vi "Computer_GUI_2.vi"(11 "GUI_cluster":T1={"Sub Panel"=refnum, "GUIdevice"="Bella_LP_Mode", "CtlRef"=refnum, "user event out"=refnum}) -> ()   [LabVIEW 2011]
uses:
  GUI_Template/GUI_master/tcp_new_data_event.ctl
  GUI_Template/GUI_master/tcp new data cluster.ctl
  Controls/GUI_cluster.ctl
  Controls/eventtypdef.ctl
panel:
  out "tcp data event":T2
  out "GUIdevice 1":string="Bella_LP_Mode"
  in  "stop":bool
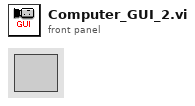
[diagram p1: front panel]
types:
  T1 = typedef "GUI_cluster.ctl" = cluster{"Sub Panel":refnum<vi>, "GUIdevice":string, "CtlRef":refnum<vi>, "user event out":refnum<user-event>}
  T2 = typedef "tcp_new_data_event.ctl" = refnum<user-event>
  T3 = typedef "eventtypdef.ctl" = cluster{"label":string, "Sub Panel":refnum<vi>, "CtlRef":refnum<vi>, "This VI":refnum<vi>}
  T4 = typedef "tcp new data cluster.ctl" = cluster{"EventEnum":enum16{"new data", "connection status update"}, "Device name":string}
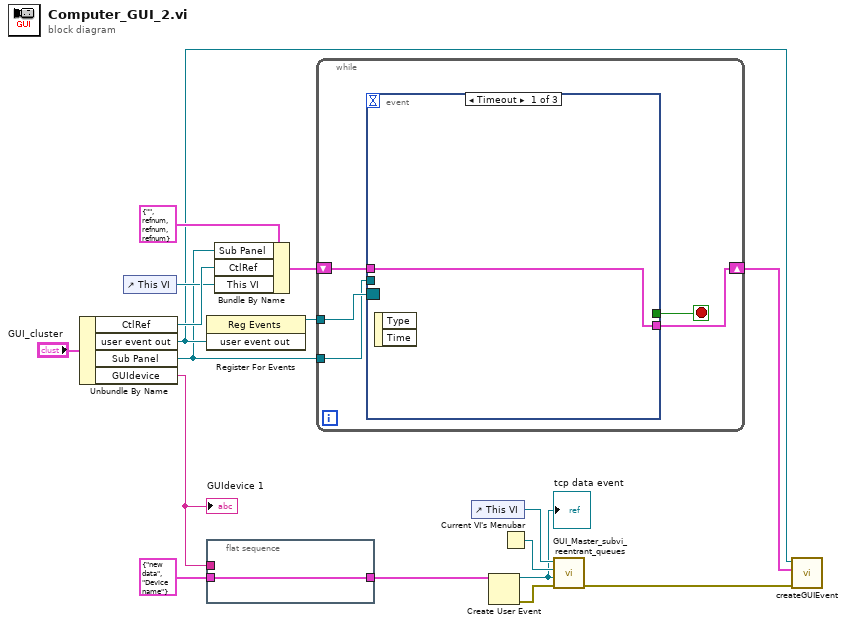
[diagram p0: block diagram]
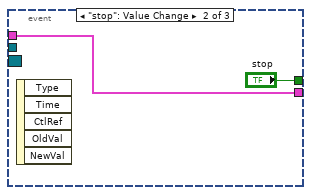
[diagram p2: hidden frame]
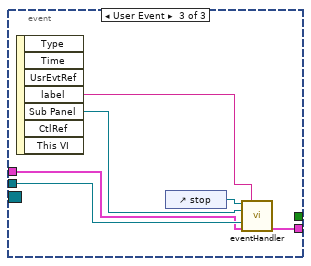
[diagram p3: hidden frame]
diagram:
  n1 = Unbundle By Name("GUI_cluster") -> ("CtlRef"=w9:refnum<vi>, "user event out"=w4:refnum<user-event>, "Sub Panel"=w2:refnum<vi>, "GUIdevice"=w7:string)
  "GUIdevice 1" <- w7
  n2 = control-ref of="This VI"() -> (w8:refnum<vi>)
  n3 = register-events(w4) -> (reference out=w3:refnum<event-registration>)  [unwired: 2 in, 1 out]
  n4 = flat-sequence {
    tunnel: T4 {"EventEnum"=enum."new data", "Device name"="Device name"} ("New Event") -> [w18]
    tunnel: [w18] -> w10
    tunnel: w7 -> [_]
    frame #0 {
    }
  }
  n5 = Bundle By Name(cluster=T3 {"label"="", "Sub Panel"=refnum, "CtlRef"=refnum, "This VI"=refnum} ("event data"), "Sub Panel"=w2, "CtlRef"=w9, "This VI"=w8) -> (w5:T3)
  n6 = while {
    shift-right: [w21] -> w1
    shift-left: w5 -> [w22]
    tunnel: w3 -> [w20]
    tunnel: w2 -> [w19]
    stop <- w23 stop-if-true
    n7 = event shown="[0] Timeout" {
      selector: w20 -> [_ _ _]
      dyn-events: _ -> [_ _ _]
      timeout: _ -> [_ _ _]
      tunnel: [_ "stop" _] -> w23
      tunnel: w22 -> [w24 w25 w29]
      tunnel: [w24 w25 w28] -> w21
      tunnel: w19 -> [_ _ w30]
      event Timeout {
        n8 = event-data() -> ()  [unwired: 1 in, 2 out]
      }
      event "stop": Value Change {
        n9 = event-data() -> ()  [unwired: 1 in, 5 out]
      }
      event User Event {
        n10 = event-data() -> ("label"=w27:string, "Sub Panel"=w31:refnum<vi>)  [unwired: 1 in, 5 out]
        n11 = control-ref of="stop"() -> (w32:refnum<vi>)
        n12 = call "eventHandler.vi"("Boolean in"=w32, "label"=w27, "Sub Panel 2"=w31, "Sub Panel"=w30, "event data in"=w29) -> ("event data out"=w28:T3)  [unwired: 10 in]
      }
    }
  }
  n13 = control-ref of="This VI"() -> (w17:refnum<vi>)
  n14 = Create User Event(user event datatype=w10) -> (user event=w14:refnum<user-event>, error out=w15:errorcluster)  [unwired: 1 in]
  "tcp data event" <- w14
  n15 = Current VI's Menubar() -> (w16:refnum<k9>)
  n16 = call "GUI_Master_subvi_reentrant_queues.vi"("error in (no error)"=w15, "tcp data event"=w14, "Caller menu reference"=w16, "Caller VI ref"=w17) -> ("error out"=w6:errorcluster)  [unwired: 7 in]
  n17 = call "createGUIEvent.vi"("error in (no error)"=w6, "event data"=w1, "User Event in"=w4) -> ()  [unwired: 9 in]
